vi "Main.vi"   [LabVIEW 2017, in "Command Pattern Demo.lvclass"]
uses:
  Command Pattern Demo.lvclass
  Stock Class/Stock.lvclass
  BuyStock Class/BuyStock.lvclass
  C:/Users/fflores/Documents/LabVIEW-Open-Projects/LabIVEW OOP Design Patterns/Command Pattern/Order Class/Order.lvclass
  SellStock Class/SellStock.lvclass
  Broker Class/Broker.lvclass
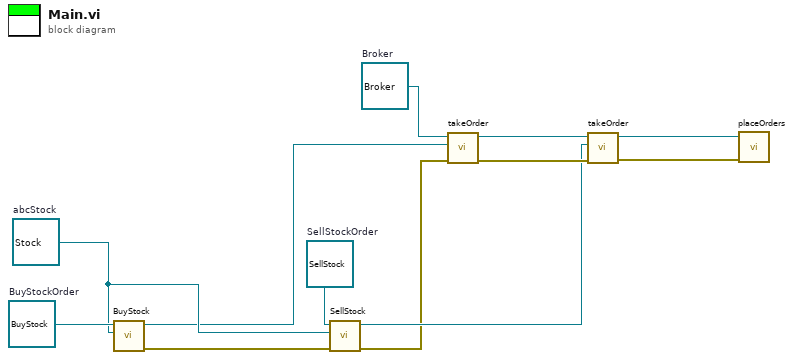
[diagram p0: block diagram]
diagram:
  w7 = refnum<class "Broker.lvclass"> refnum  # Broker
  w12 = refnum<class "SellStock.lvclass"> refnum  # SellStockOrder
  w11 = refnum<class "BuyStock.lvclass"> refnum  # BuyStockOrder
  w10 = refnum<class "Stock.lvclass"> refnum  # abcStock
  n1 = call "BuyStock.vi"("Stock.lvclass"=w10, "BuyStock in"=w11) -> ("error out"=w4:errorcluster, "BuyStock out"=w6:refnum<class "BuyStock.lvclass">)  [unwired: 8 in]
  n2 = call "SellStock.vi"("error in (no error)"=w4, "Stock.lvclass"=w10, "SellStock in"=w12) -> ("error out"=w3:errorcluster, "SellStock out"=w5:refnum<class "SellStock.lvclass">)  [unwired: 7 in]
  n3 = call "takeOrder.vi"("error in (no error)"=w3, "Order.lvclass"=w6, "Broker in"=w7) -> ("error out"=w8:errorcluster, "Broker out"=w9:refnum<class "Broker.lvclass">)  [unwired: 7 in]
  n4 = call "takeOrder.vi"("error in (no error)"=w8, "Order.lvclass"=w5, "Broker in"=w9) -> ("error out"=w1:errorcluster, "Broker out"=w2:refnum<class "Broker.lvclass">)  [unwired: 7 in]
  n5 = call "placeOrders.vi"("error in (no error)"=w1, "Broker in"=w2) -> ()  [unwired: 8 in, 2 out]
